vi "main.vi"() -> ()   [LabVIEW 2013]
doc: "This.vi will programmatically open and run That.vi, using VI Server. Unlike a subVI, That.vi will run independently of This.vi, with control being returned to This.vi immediately.\n\nNote: You would only make a call to That.vi once (i.e., don't use a while loop to control it), unless you know that it has stopped running, in which case, you can call it again."
uses:
  Global 1.vi
panel:
  in  "Cycles Requested":i32=50
  out "Last Beat":bool
  out "Heartbeat count":i32
  out "Task running":bool
  out "Heart rate":dbl format="%#_3g"
  out "Task heartbeat":bool
  out "Command sent":bool
  out "Last Time Stamp":timestamp
  out "Chart from task":dbl(graph)
  out "Task info / error out":errorcluster
  in  "task name":string="task1.vi"
  in  "Abort Task1":bool
  out "Task Random #":dbl format="%#_4g"
  # "Main.vi will programmatically open and run task1.vi, using VI Server.  Unlike a subVI, task1.vi will run independently of main.vi, \nwith control being returned to main.vi immediately."
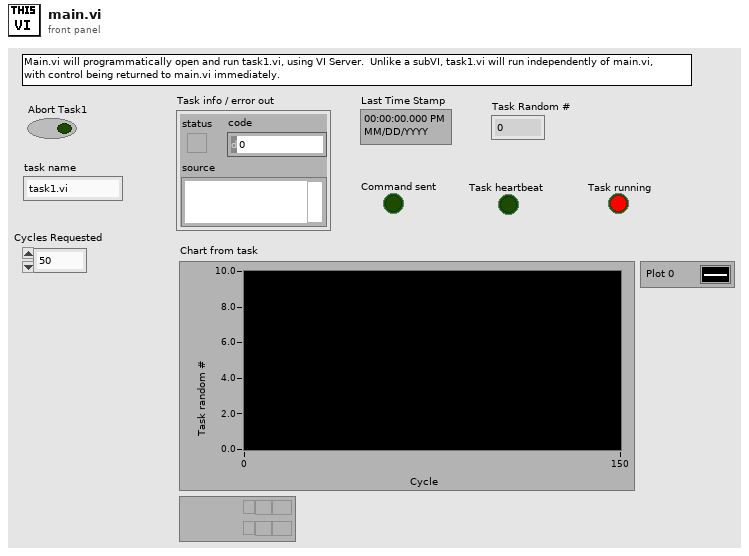
[diagram p1: front panel]
types:
  T1 = enum32{"Bad", "Idle", "Run top level", "Running"}
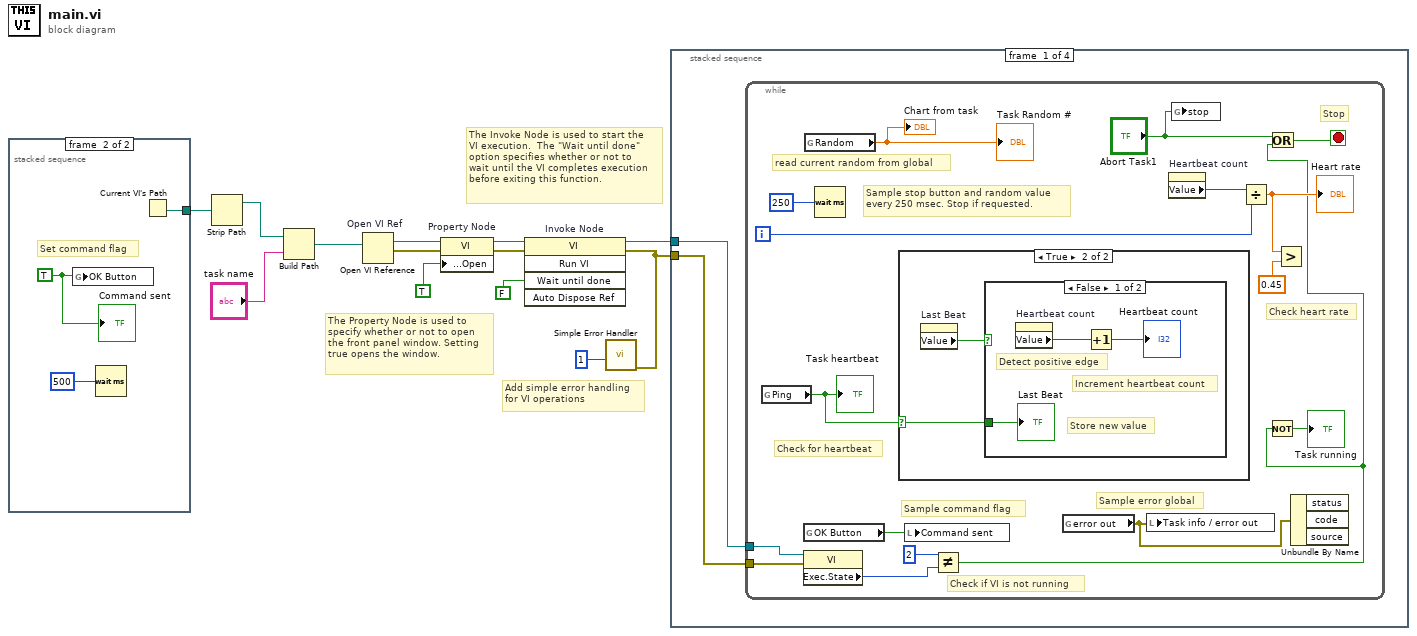
[diagram p0: block diagram]
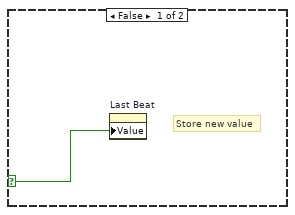
[diagram p2: hidden frame]
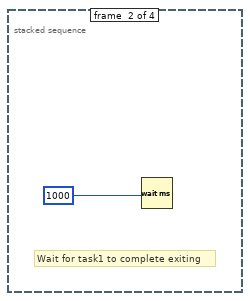
[diagram p4: hidden frame]
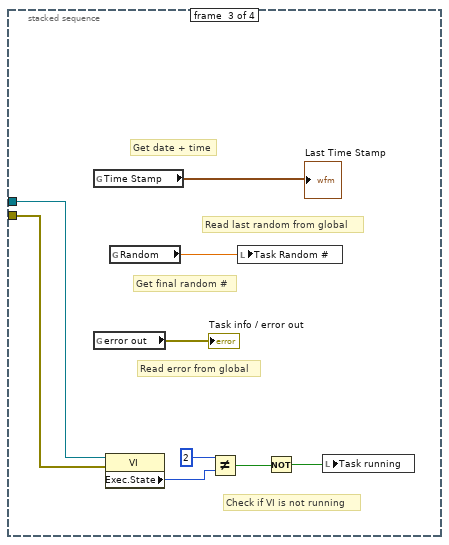
[diagram p5: hidden frame]
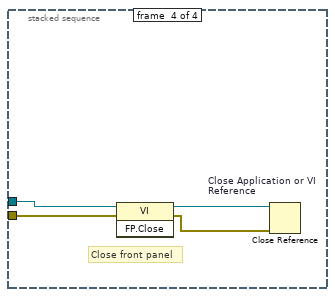
[diagram p6: hidden frame]
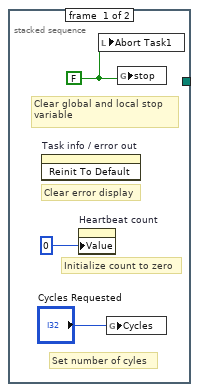
[diagram p7: hidden frame]
diagram:
  # "Add simple error handling\nfor VI operations"
  # "The Invoke Node is used to start the \nVI execution.  The \"Wait until done\" \noption specifies whether or not to \nwait until the VI completes execution\nbefore exiting this function."
  # "The Property Node is used to \nspecify whether or not to open \nthe front panel window. Setting\ntrue opens the window."
  n1 = stacked-sequence {
    tunnel: [_ w19] -> w7
    frame #0 {
      w16 = FALSE
      # "Set number of cyles"
      # "Initialize count to zero"
      # "Clear error display"
      # "Clear global and local stop \nvariable"
      n2 = invoke on="Task info / error out" class="Clust (strict)" method="Reinit To Default"() -> ()  [unwired: 3 in, 3 out]
      n3 = property on="Heartbeat count" class="DigNum (strict)"("Value"=0) -> ()  [unwired: 2 in, 2 out]
      n4 = local write "Abort Task1"(w16) -> ()
      n5 = global write "Global 1.vi" "Cycles"("Cycles Requested") -> ()
      n6 = global write "Global 1.vi" "stop"(w16) -> ()
    }
    frame #1 {
      w18 = TRUE ("Front Panel.Open")
      # "Set command flag"
      n7 = global write "Global 1.vi" "OK Button"(w18) -> ()
      n8 = Wait (ms)(milliseconds to wait=500) -> ()  [unwired: 1 out]
      n9 = Current VI's Path() -> (path=w19:path)
      "Command sent" <- w18
    }
  }
  n10 = Strip Path(path=w7) -> (stripped path=w9:path)  [unwired: 1 out]
  n11 = Build Path(base path=w9, name or relative path="task name") -> (appended path=w10:path)
  n12 = Open VI Reference "Open VI Ref"(vi path=w10) -> (vi reference=w13:refnum<vi>, error out=w6:errorcluster)  [unwired: 5 in]
  n13 = property on="Property Node" class="VI"(reference=w13, error in=w6, "Front Panel Window:Open"=TRUE ("Front Panel.Open")) -> (reference out=w2:refnum<vi>, error out=w1:errorcluster)
  n14 = invoke on="Invoke Node" class="VI" method="Run VI"(reference=w2, error in=w1, "Wait until done"=FALSE) -> (reference out=w3:refnum<vi>, error out=w4:errorcluster)  [unwired: 2 in, 3 out]
  n15 = call <vilib>:"Simple Error Handler.vi"("type of dialog (OK msg:1)"=1, "error in (no error)"=w4) -> ()  [unwired: 3 in, 5 out]
  n16 = stacked-sequence {
    tunnel: w4 -> [w20 _ w46 w57]
    tunnel: w3 -> [w21 _ w47 w58]
    frame #0 {
      n17 = while {
        tunnel: w21 -> [w27]
        tunnel: w20 -> [w26]
        i -> [w33]
        stop <- w28 stop-if-true
        # "Check if VI is not running"
        # "Sample error global"
        # "Sample command flag"
        # "Check for heartbeat"
        # "Check heart rate"
        # "Stop"
        # "read current random from global"
        # "Sample stop button and random value\nevery 250 msec. Stop if requested."
        n18 = global read "Global 1.vi" "Ping"() -> (w36:bool)
        "Task heartbeat" <- w36
        n19 = global read "Global 1.vi" "OK Button"() -> (w31:bool)
        n20 = property class="VI"(reference=w27, error in=w26) -> ("Exec.State"=w24:T1)  [unwired: 2 out]
        n21 = global read "Global 1.vi" "Random"() -> (→"Task Random #" →"Chart from task":dbl)
        n22 = Wait (ms)(milliseconds to wait=250) -> ()  [unwired: 1 out]
        n23 = case shown="True" w36 {
          selector: w36 -> [w39 w40]
          frame False {
            # "Store new value"
            n24 = property on="Last Beat" class="Bool (strict)"("Value"=w39) -> ()  [unwired: 2 in, 2 out]
          }
          frame True {
            n25 = property on="Last Beat" class="Bool (strict)"() -> ("Value"=w41:bool)  [unwired: 2 in, 2 out]
            n26 = case shown="False" w41 {
              tunnel: w40 -> [w42 _]
              frame False {
                # "Store new value"
                # "Detect positive edge"
                # "Increment heartbeat count"
                n27 = property on="Heartbeat count" class="DigNum (strict)"() -> ("Value"=w44:i32)  [unwired: 2 in, 2 out]
                n28 = Increment(x=w44) -> (x+1=→"Heartbeat count":i32)
                "Last Beat" <- w42
              }
              frame True {
              }
            }
          }
        }
        n29 = local write "Command sent"(w31) -> ()
        n30 = Not Equal?(x=2, y=w24) -> (x != y?=w22:bool)
        n31 = global read "Global 1.vi" "error out"() -> (w30:errorcluster)
        n32 = local write "Task info / error out"(w30) -> ()
        n33 = property on="Heartbeat count" class="DigNum (strict)"() -> ("Value"=w32:i32)  [unwired: 2 in, 2 out]
        n34 = global write "Global 1.vi" "stop"("Abort Task1") -> ()
        n35 = Divide(x=w32, y=w33) -> (x/y=w34:dbl)
        "Heart rate" <- w34
        n36 = Not(x=w22) -> (.not. x?=→"Task running":bool)
        n37 = Or(x="Abort Task1", y=w22) -> (x .or. y?=w28:bool)
        n38 = Greater?(x=w34, y=0.45) -> ()  [unwired: 1 out]
        n39 = Unbundle By Name(w30) -> ()  [unwired: 3 out]
      }
    }
    frame #1 {
      # "Wait for task1 to complete exiting"
      n40 = Wait (ms)(milliseconds to wait=1000) -> ()  [unwired: 1 out]
    }
    frame #2 {
      # "Check if VI is not running"
      # "Get date + time"
      # "Read error from global"
      # "Read last random from global"
      # "Get final random #"
      n41 = global read "Global 1.vi" "Time Stamp"() -> (→"Last Time Stamp":timestamp)
      n42 = global read "Global 1.vi" "error out"() -> (→"Task info / error out":errorcluster)
      n43 = property class="VI"(reference=w47, error in=w46) -> ("Exec.State"=w50:T1)  [unwired: 2 out]
      n44 = global read "Global 1.vi" "Random"() -> (w54:dbl)
      n45 = Not Equal?(x=2, y=w50) -> (x != y?=w49:bool)
      n46 = local write "Task Random #"(w54) -> ()
      n47 = Not(x=w49) -> (.not. x?=w48:bool)
      n48 = local write "Task running"(w48) -> ()
    }
    frame #3 {
      # "Close front panel"
      n49 = invoke class="VI" method="FP.Close"(reference=w58, error in=w57) -> (reference out=w56:refnum<vi>, error out=w55:errorcluster)  [unwired: 1 in, 1 out]
      n50 = Close Reference "Close Application or VI Reference"(reference=w56, error in (no error)=w55) -> ()  [unwired: 1 out]
    }
  }
